vi "DLS ERD Parse.vi"(11 "ERD Data Out":T1[](array[typedef]) {"ERD Number" format="%.0x"}) -> (3 "DLS ERD Data 2":T2)   [LabVIEW 2016, in "2015 VA Washer.lvlib"]
uses:
  Projects/2015 VA Washer.lvlib
  Control/DLS ERD Data.ctl
  Common/LabVIEW GEA2 Toolkit/LabVIEW_GEA2_Toolkit.lvlibp/type defs/ERD Read Data Out.ctl
  Common/LabVIEW GEA2 Toolkit/LabVIEW_GEA2_Toolkit.lvlibp
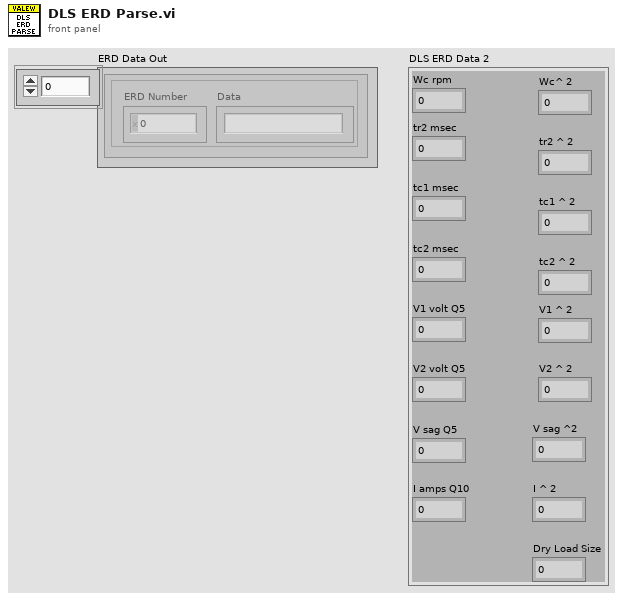
[diagram p1: front panel]
types:
  T1 = typedef "LabVIEW_GEA2_Toolkit.lvlibp/ERD Read Data Out.ctl" = cluster{"ERD Number":u16, "Data":string}
  T2 = typedef "2015 VA Washer.lvlib/DLS ERD Data.ctl" = cluster{"Wc rpm":dbl, "tr2 msec":dbl, "tc1 msec":dbl, "tc2 msec":dbl, "V1 volt Q5":dbl, "V2 volt Q5":dbl, "I amps Q10":dbl, "Wc^ 2":dbl, "tr2 ^ 2":dbl, "tc1 ^ 2":dbl, "tc2 ^ 2":dbl, "V1 ^ 2":dbl, "V2 ^ 2":dbl, "I ^ 2":dbl, "V sag Q5":dbl, "V sag ^2":dbl, "Dry Load Size":dbl}
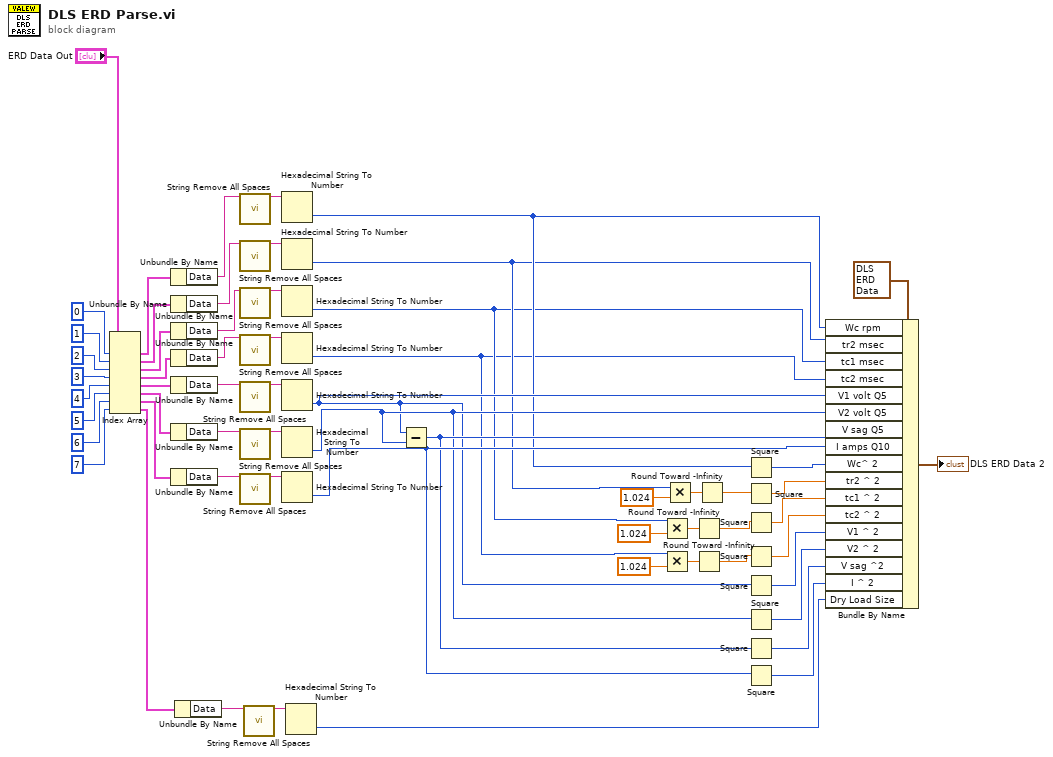
[diagram p0: block diagram]
diagram:
  n1 = Index Array(array="ERD Data Out", index #1=0 ("index"), index #2=1 ("index"), index #3=2 ("index"), index #4=3 ("index"), index #5=4 ("index"), index #6=5 ("index"), index #7=6 ("index"), index #8=7 ("index")) -> (element #1=w14:T1, element #2=w22:T1, element #3=w23:T1, element #4=w24:T1, element #5=w25:T1, element #6=w26:T1, element #7=w27:T1, element #8=w29:T1)
  n2 = Unbundle By Name(w14) -> ("Data"=w31:string)
  n3 = Unbundle By Name(w22) -> ("Data"=w39:string)
  n4 = Unbundle By Name(w23) -> ("Data"=w40:string)
  n5 = Unbundle By Name(w24) -> ("Data"=w41:string)
  n6 = Unbundle By Name(w25) -> ("Data"=w42:string)
  n7 = Unbundle By Name(w26) -> ("Data"=w43:string)
  n8 = Unbundle By Name(w27) -> ("Data"=w44:string)
  n9 = Unbundle By Name(w29) -> ("Data"=w45:string)
  n10 = call "String Remove All Spaces.vi"("Input String"=w31) -> ("Spaces Removed"=w30:string)  [unwired: 13 in, 1 out]
  n11 = call "String Remove All Spaces.vi"("Input String"=w39) -> ("Spaces Removed"=w32:string)  [unwired: 13 in, 1 out]
  n12 = call "String Remove All Spaces.vi"("Input String"=w40) -> ("Spaces Removed"=w33:string)  [unwired: 13 in, 1 out]
  n13 = call "String Remove All Spaces.vi"("Input String"=w41) -> ("Spaces Removed"=w34:string)  [unwired: 13 in, 1 out]
  n14 = call "String Remove All Spaces.vi"("Input String"=w42) -> ("Spaces Removed"=w35:string)  [unwired: 13 in, 1 out]
  n15 = call "String Remove All Spaces.vi"("Input String"=w43) -> ("Spaces Removed"=w36:string)  [unwired: 13 in, 1 out]
  n16 = call "String Remove All Spaces.vi"("Input String"=w44) -> ("Spaces Removed"=w37:string)  [unwired: 13 in, 1 out]
  n17 = call "String Remove All Spaces.vi"("Input String"=w45) -> ("Spaces Removed"=w38:string)  [unwired: 13 in, 1 out]
  n18 = Hexadecimal String To Number(string=w30) -> (number=w48:u32)  [unwired: 2 in, 1 out]
  n19 = Hexadecimal String To Number(string=w32) -> (number=w9:u32)  [unwired: 2 in, 1 out]
  n20 = Hexadecimal String To Number(string=w33) -> (number=w5:u32)  [unwired: 2 in, 1 out]
  n21 = Hexadecimal String To Number(string=w34) -> (number=w1:u32)  [unwired: 2 in, 1 out]
  n22 = Hexadecimal String To Number(string=w35) -> (number=w57:u32)  [unwired: 2 in, 1 out]
  n23 = Hexadecimal String To Number(string=w36) -> (number=w58:u32)  [unwired: 2 in, 1 out]
  n24 = Hexadecimal String To Number(string=w37) -> (number=w60:u32)  [unwired: 2 in, 1 out]
  n25 = Hexadecimal String To Number(string=w38) -> (number=w47:u32)  [unwired: 2 in, 1 out]
  n26 = Subtract(x=w57, y=w58) -> (x-y=w59:u32)
  n27 = Multiply(x=w5, y=1.024) -> (x*y=w7:dbl)
  n28 = Multiply(x=w1, y=1.024) -> (x*y=w3:dbl)
  n29 = Multiply(x=w9, y=1.024) -> (x*y=w11:dbl)
  n30 = Round Toward -Infinity(1:w7) -> (0:w6:dbl)
  n31 = Round Toward -Infinity(1:w3) -> (0:w2:dbl)
  n32 = Round Toward -Infinity(1:w11) -> (0:w10:dbl)
  n33 = Square(x=w48) -> (x^2=w49:u32)
  n34 = Square(x=w10) -> (x^2=w50:dbl)
  n35 = Square(x=w6) -> (x^2=w51:dbl)
  n36 = Square(x=w2) -> (x^2=w52:dbl)
  n37 = Square(x=w57) -> (x^2=w53:u32)
  n38 = Square(x=w58) -> (x^2=w54:u32)
  n39 = Square(x=w59) -> (x^2=w55:u32)
  n40 = Square(x=w60) -> (x^2=w56:u32)
  n41 = Bundle By Name(cluster=T2 {"Wc rpm"=0.0, "tr2 msec"=0.0, "tc1 msec"=0.0, "tc2 msec"=0.0, "V1 volt Q5"=0.0, "V2 volt Q5"=0.0, "I amps Q10"=0.0, "Wc^ 2"=0.0, "tr2 ^ 2"=0.0, "tc1 ^ 2"=0.0, "tc2 ^ 2"=0.0, "V1 ^ 2"=0.0, "V2 ^ 2"=0.0, "I ^ 2"=0.0, "V sag Q5"=0.0, "V sag ^2"=0.0, "Dry Load Size"=0.0} ("DLS ERD Data 2"), "Wc rpm"=w48, "tr2 msec"=w9, "tc1 msec"=w5, "tc2 msec"=w1, "V1 volt Q5"=w57, "V2 volt Q5"=w58, "V sag Q5"=w59, "I amps Q10"=w60, "Wc^ 2"=w49, "tr2 ^ 2"=w50, "tc1 ^ 2"=w51, "tc2 ^ 2"=w52, "V1 ^ 2"=w53, "V2 ^ 2"=w54, "V sag ^2"=w55, "I ^ 2"=w56, "Dry Load Size"=w47) -> (→"DLS ERD Data 2":T2)
